vi "InitDigitizer.vi"(0 "Digitizer ID":T2 caption="RIO Device", 1 "Delay After Trig (us)":dbl, 2 "Sampling Frequency":dbl, 9 "Trigger Type":enum8{"Software", "Data Edge"}(ring), 11 "Record Size":u32, 12 "Trigger Level (V)":dbl) -> (6 "TIS Configured?":bool, 8 "Clocking Configured?":bool, 10 "Default Configured?":bool, 14 "Digitizer Info":T1, 15 "Error out":errorcluster)   [LabVIEW 2018]
uses:
  <vilib>/userdefined/High Color/nirio_resource_hc.ctl
  Controls/DigitizerInfo.ctl
  FPGA/Digitizer 5772/Controls/TIS Mode.ctl
panel:
  out "range (Vpp)":dbl
  out "Num of Elements":u16
  # "Keep it a multi of 8"
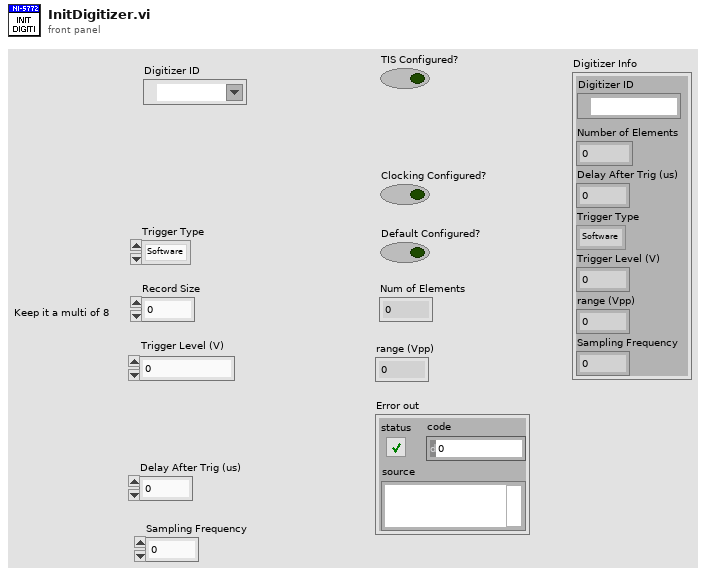
[diagram p1: front panel]
types:
  T1 = typedef "DigitizerInfo.ctl" = cluster{"Digitizer ID":T2, "Number of Elements":u16, "Delay After Trig (us)":dbl, "Trigger Type":enum8{"Software", "Data Edge"}, "Trigger Level (V)":dbl, "range (Vpp)":dbl, "Sampling Frequency":dbl}
  T2 = typedef "nirio_resource_hc.ctl" = tag
  T3 = enum8{"Internal Clock PLL Off", "Internal Clock PLL On (REF IN)", "External Clock (CLK_IN)", "Internal Clock PLL On (IoModSyncClk)"}
  T4 = typedef "TIS Mode.ctl" = u16
  T5 = cluster{"Digitizer ID":T2, "Number of Elements":u16, "Delay After Trig (us)":dbl, "Trigger Type":enum8{"Software", "Data Edge"}, "Trigger Level (V)":dbl, "range (Vpp)":dbl, "Sampling Frequency":dbl}
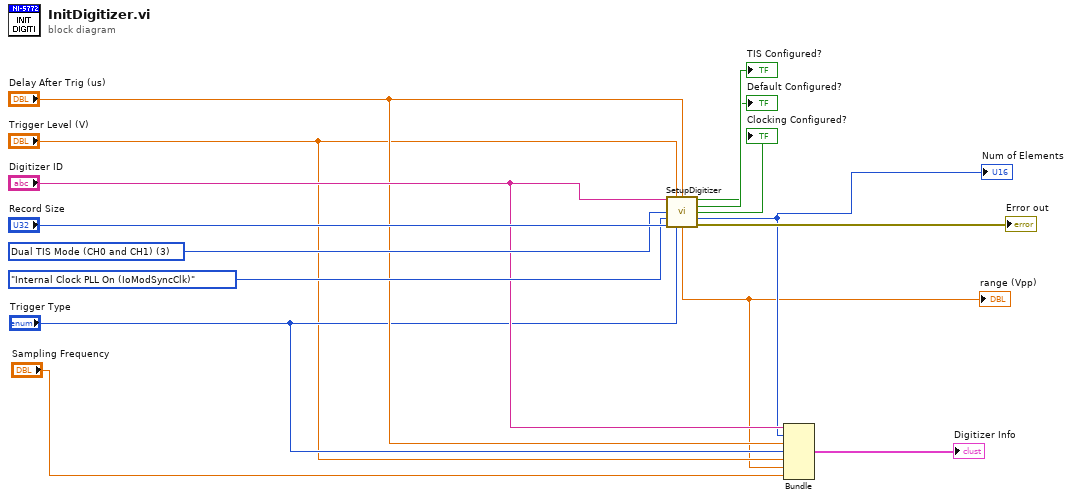
[diagram p0: block diagram]
diagram:
  w14 = T4 3 items=["TIS Mode (CH0 Only)"=1, "TIS Mode (CH1 Only)"=2, "Dual TIS Mode (CH0 and CH1)"=3] ("TIS Mode")
  n1 = call "SetupDigitizer.vi"("RIO Resource`"="Digitizer ID", "Trigger Level (V)"="Trigger Level (V)", "Delay after Trig (us)"="Delay After Trig (us)", "Record Size"="Record Size", "TIS Mode"=w14, "Clock Source"=T3."Internal Clock PLL On (IoModSyncClk)", "Trigger Type"="Trigger Type") -> ("Default Configured?"=→"Default Configured?":bool, "TIS Configured?"=→"TIS Configured?":bool, "Clocking Option Configured?"=→"Clocking Configured?":bool, "Number of Elements"=w7:u16, "range (Vpp)"=w3:dbl, "error out"=→"Error out":errorcluster)  [unwired: 3 in]
  "Num of Elements" <- w7
  "range (Vpp)" <- w3
  n2 = Bundle("Digitizer ID"="Digitizer ID", "Number of Elements"=w7, "Delay After Trig (us)"="Delay After Trig (us)", "Trigger Type"="Trigger Type", "Trigger Level (V)"="Trigger Level (V)", "range (Vpp)"=w3, "Sampling Frequency"="Sampling Frequency") -> (→"Digitizer Info":T5)  [unwired: 1 in]
